vi "Initialize TCPIP.vi"(8 "error in (no error)":errorcluster, 9 "Read Timeout (100ms)":u32=100, 11 "VISA resource name in":refnum<visa-resource-name>) -> (0 "error out":errorcluster, 3 "VISA resource name out":refnum<visa-resource-name>)   [LabVIEW 2020, in "Zaber A Series.lvlib"]
doc: "Establishes communication with a Zaber device over TCP/IP. Call this VI before calling other instrument driver VIs for this instrument. You need to call the Initialize VI only once at the beginning of an application, or again after using the Close VI. i"
uses:
  Zaber A Series.lvlib
panel:
  # "(c) 2017-2021 Zaber Technologies.  ALL RIGHTS RESERVED."
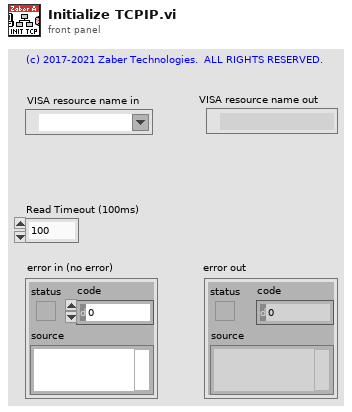
[diagram p1: front panel]
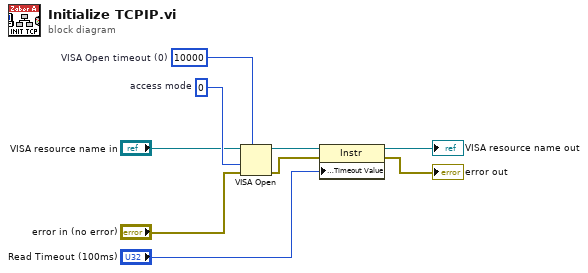
[diagram p0: block diagram]
diagram:
  w7 = u32 10000  # VISA Open timeout (0)
  w9 = u32 0  # access mode
  n1 = VISA Open(timeout (0)=w7, access mode=w9, error in (no error)="error in (no error)", VISA resource name="VISA resource name in") -> (VISA resource name=w5:refnum<visa-resource-name>, error out=w6:errorcluster)  [unwired: 1 in]
  n2 = property class="Instr"(reference=w5, error in=w6, "General Settings:Timeout Value"="Read Timeout (100ms)") -> (reference out=→"VISA resource name out":refnum<visa-resource-name>, error out=→"error out":errorcluster)
